vi "OpenTypedef.vi"(6 "Mouse Position":T1, 7 "User VI Ref":refnum<vi>, 8 "Is Multi-select?":bool, 9 "Remaining Items":refnum<vi>[](array[refnum]), 10 "Affected Items":T8, 11 "Menu Refnum":refnum<k9>) -> (3 "Menu Items To Add":T2[](array[typedef]))   [LabVIEW 2020]
doc: "This VI is part of a plug-in for modifying the LabVIEW shortcut menus. This is the builder VI which is called when the shortcut menu is built. It tells LabVIEW which shortcut menu items to add to the menu."
uses:
  <resource>/plugins/PopupMenus/support/Checkmark Status.ctl
  <resource>/plugins/PopupMenus/support/Relative Position.ctl
  <resource>/plugins/PopupMenus/support/Position In Menu.ctl
  <resource>/plugins/PopupMenus/support/Transaction Control.ctl
  <resource>/plugins/PopupMenus/support/Shortcut Menu Item Definition.ctl
  <resource>/plugins/PopupMenus/support/Enabled Menu Item Status.ctl
  <vilib>/Utility/Data Type/Type Definitions/Data Type.ctl
  <vilib>/Utility/Data Type/NI_Data Type.lvlib
  OpenTypedef.ctl
  <vilib>/Utility/miscctls.llb/LVPositionTypeDef.ctl
panel:
  # "Rules a popup plug-in must follow:\n* This VI's file name must match the file name of the LLB -- only the file extensions should be different.\n* This VI must have debugging disabled or it will be ignored as a plug-in.\n* For all menu items, \"tag suffix + file name of this VI\" must be less than 240 characters.\n* You can disconnect the \"Affected Items\" from the typedef to make the plug-in load faster. The typedef is only there to assist you in keeping this VI and the execution VI using to the same type.\n* All controls on this panel except \"Affected Items\" are locked to prevent accidental edits. Do not change the types or the names of controls other than the elements inside the \"Affected Items\" cluster.\n* See Context Help for more information on the individual controls."
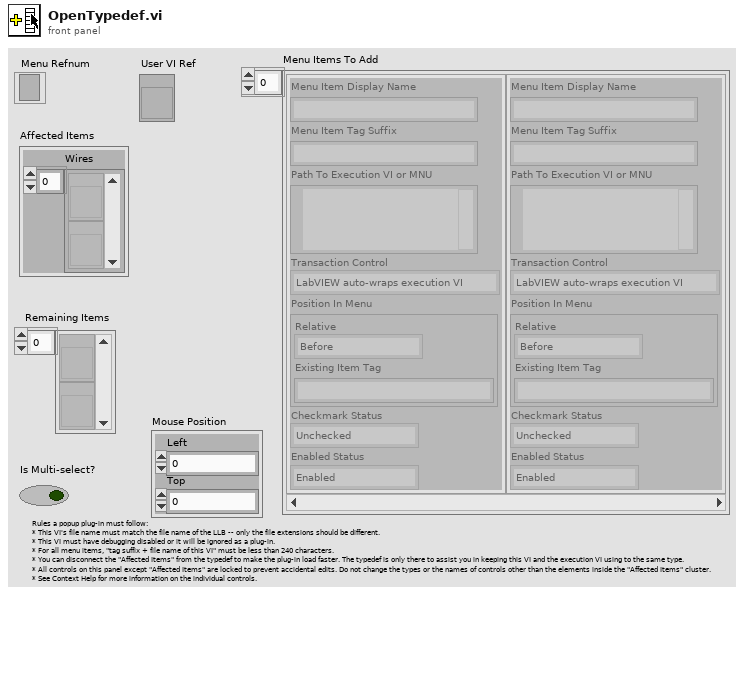
[diagram p1: front panel]
types:
  T1 = typedef "LVPositionTypeDef.ctl" = cluster{"Left":i32, "Top":i32}
  T2 = typedef "Shortcut Menu Item Definition.ctl" = cluster{"Menu Item Display Name":string, "Menu Item Tag Suffix":string, "Path To Execution VI or MNU":path, "Transaction Control":T3, "Position In Menu":T4, "Checkmark Status":T6, "Enabled Status":T7}
  T3 = typedef "Transaction Control.ctl" = enum8{"LabVIEW auto-wraps execution VI", "Execution VI will define if needed"}
  T4 = typedef "Position In Menu.ctl" = cluster{"Relative":T5, "Existing Item Tag":string}
  T5 = typedef "Relative Position.ctl" = enum8{"Before", "Instead of", "After", "Into Submenu"}
  T6 = typedef "Checkmark Status.ctl" = enum8{"Unchecked", "Checked"}
  T7 = typedef "Enabled Menu Item Status.ctl" = enum8{"Enabled", "Disabled"}
  T8 = typedef "OpenTypedef.ctl" = cluster{"Wires":refnum<vi>[]}
  T9 = typedef "NI_Data Type.lvlib/Data Type.ctl" = enum8{"Invalid Type", "Void", "I8", "I16", "I32", "I64", "U8", "U16", "U32", "U64", "Single Float", "Double Float", "Extended Float", "Single Complex", "Double Complex", "Extended Complex", "Enum U8", "Enum U16", "Enum U32", "Enum U64", "Single Float With Unit", "Double Float With Unit", "Extended Float With Unit", "Single Complex with Unit", "Double Complex with Unit", "Extended Complex with Unit", "Boolean", "String", "Path", "Picture", "Tag", "Array", "Cluster", "Variant", "LV Variant", "Waveform", "Timestamp", "Digital Waveform", "Digital Data", "ExpressData", "Refnum", "External Data", "VI", "Poly VI", "LabVIEW Class Instance", "Fixed Point", "Set Collection", "Map Collection"}
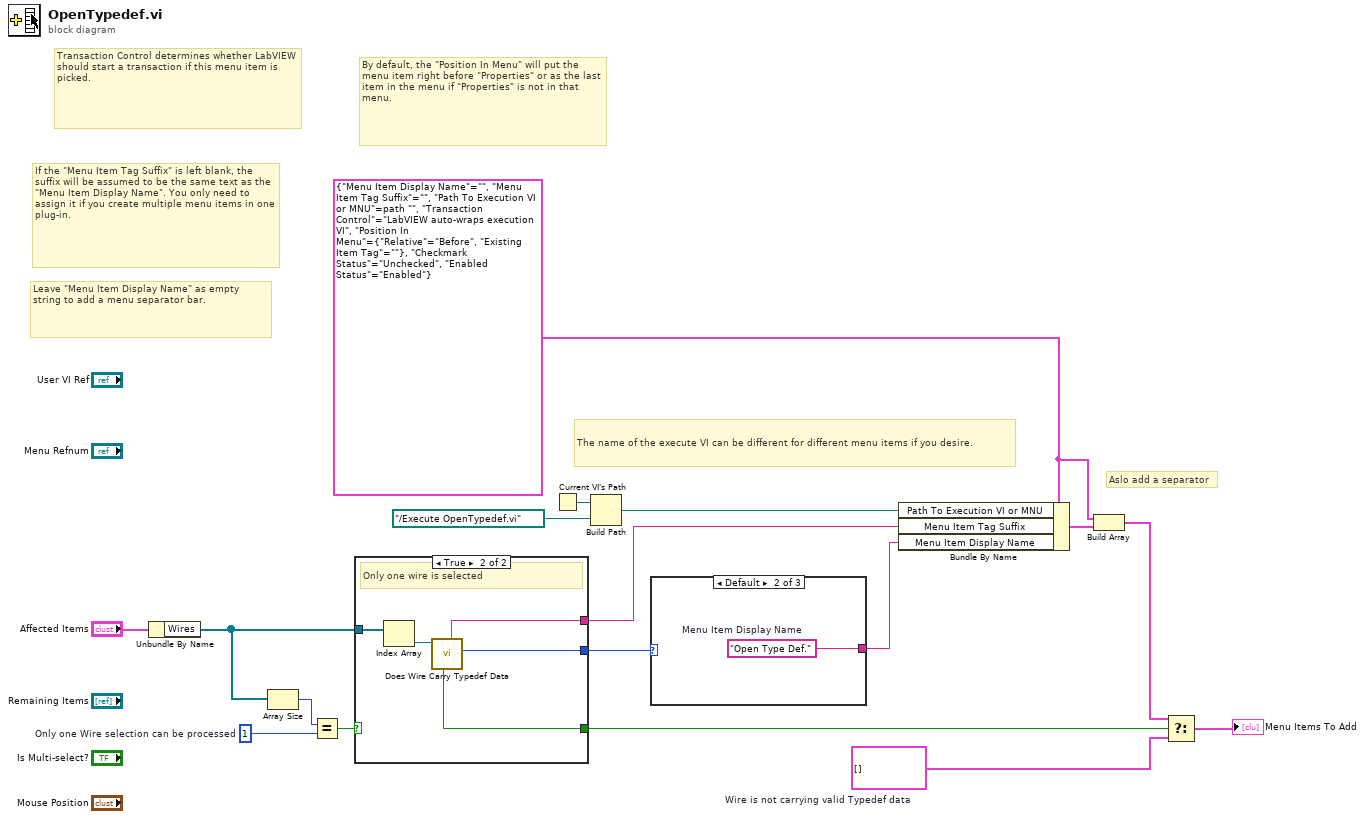
[diagram p0: block diagram]
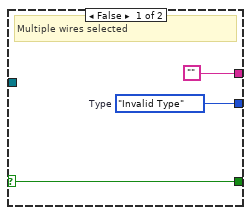
[diagram p2: hidden frame]
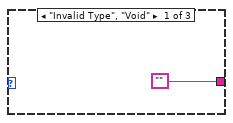
[diagram p3: hidden frame]
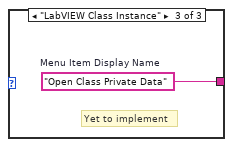
[diagram p4: hidden frame]
diagram:
  w5 = T2[] []  # Wire is not carrying valid Typedef data
  w11 = 1  # Only one Wire selection can be processed
  w1 = T2 {"Menu Item Display Name"="", "Menu Item Tag Suffix"="", "Path To Execution VI or MNU"=path "", "Transaction Control"=enum."LabVIEW auto-wraps execution VI", "Position In Menu"={"Relative"=enum."Before", "Existing Item Tag"=""}, "Checkmark Status"=enum."Unchecked", "Enabled Status"=enum."Enabled"} ("Cluster")
  # "Aslo add a separator"
  # "Transaction Control determines whether LabVIEW should start a transaction if this menu item is picked."
  # "Leave \"Menu Item Display Name\" as empty string to add a menu separator bar."
  # "If the \"Menu Item Tag Suffix\" is left blank, the suffix will be assumed to be the same text as the \"Menu Item Display Name\". You only need to assign it if you create multiple menu items in one plug-in."
  # "By default, the \"Position In Menu\" will put the menu item right before \"Properties\" or as the last item in the menu if \"Properties\" is not in that menu."
  # "The name of the execute VI can be different for different menu items if you desire."
  n1 = Unbundle By Name("Affected Items") -> ("Wires"=w10:refnum<vi>[])
  n2 = Array Size(array=w10) -> (size(s)=w12:i32)
  n3 = Equal?(x=w12, y=w11) -> (x = y?=w9:bool)
  n4 = case shown="True" w9 {
    selector: w9 -> [w20 _]
    tunnel: w10 -> [_ w25]
    tunnel: [w20 w21] -> w8
    tunnel: ["" w22] -> w4
    tunnel: [w18 w23] -> w2
    frame False {
      w18 = Data_Type."Invalid Type"  # Type
      # "Multiple wires selected"
    }
    frame True {
      # "Only one wire is selected"
      n5 = Index Array(array=w25) -> (element=w24:refnum<vi>)  [unwired: 1 in]
      n6 = call "Does Wire Carry Typedef Data.vi"("Wire in"=w24) -> ("Type"=w23:T9, "Type Definition/Class Path"=w22:string, "Wire carry Typedef/Class"=w21:bool)  [unwired: 4 in, 2 out]
    }
  }
  n7 = Current VI's Path() -> (path=w14:path)
  n8 = Build Path(base path=w14, name or relative path=path "../Execute OpenTypedef.vi" ("execute path")) -> (appended path=w16:path)
  n9 = case shown="Default" w2 {
    tunnel: ["" w27 w28] -> w3
    frame "Invalid Type", "Void" {
    }
    frame Default {
      w27 = "Open Type Def."  # Menu Item Display Name
    }
    frame "LabVIEW Class Instance" {
      w28 = "Open Class Private Data"  # Menu Item Display Name
      # "Yet to implement"
    }
  }
  n10 = Bundle By Name(cluster=w1, "Path To Execution VI or MNU"=w16, "Menu Item Tag Suffix"=w4, "Menu Item Display Name"=w3) -> (w15:T2)
  n11 = Build Array(w1, w15) -> (w7:T2[])
  n12 = Select(t=w7, s=w8, f=w5) -> (s? t:f=→"Menu Items To Add":T2[])
